vi "ToscaTTL-Enqueue Control Events.vi"(0 "TTL":refnum<class "TTLController.lvclass">[](array[class]), 7 "Rxn time":dbl) -> (15 "error out":errorcluster)   [LabVIEW 2020]
uses:
  Control Classes/Base Class/TTLController.lvclass
  Control Classes/Base Class/TTLController.lvclass/TTLController.ctl
  Control Classes/Base Class/Read Name.vi
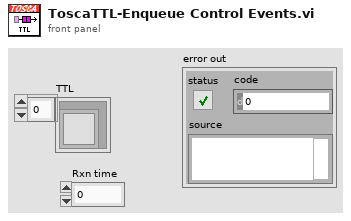
[diagram p1: front panel]
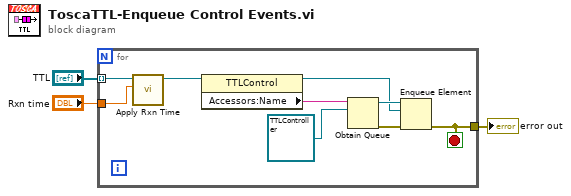
[diagram p0: block diagram]
diagram:
  n1 = for {
    tunnel: "TTL" -> [w6] mode=indexing
    tunnel: [w7] -> w2
    tunnel: "Rxn time" -> [w4]
    stop <- w7 stop-if-true
    n2 = call-dynamic "Apply Rxn Time.vi"("Trxn"=w4, "TTLControl in"=w6) -> ("TTLControl out"=w5:refnum<class "TTLController.lvclass">)  [unwired: 8 in, 1 out]
    n3 = property class="TTLControl"(reference=w5) -> (reference out=w8:refnum<class "TTLController.lvclass">, "Accessors:Name"=w12:string)  [unwired: 1 in, 1 out]
    n4 = Obtain Queue(name (unnamed)=w12, element data type=refnum<class "TTLController.lvclass"> refnum ("TTL")) -> (queue out=w9:refnum<queue>, error out=w10:errorcluster)  [unwired: 3 in, 1 out]
    n5 = Enqueue Element(queue=w9, element=w8, error in (no error)=w10) -> (error out=w7:errorcluster)  [unwired: 1 in, 2 out]
  }
  "error out" <- w2
